vi "Export Test Suite.vi"(8 "error in (no error)":errorcluster, 10 "Test Suite":T1, 11 "Node in":refnum<k20>) -> (0 "error out":errorcluster, 3 "Node out":refnum<k20>)   [LabVIEW 2013, in "JUnit for Azure Pipelines.lvclass"]
uses:
  JUnit for Azure Pipelines.lvclass
  Test Suite.ctl
  Test Case.ctl
  Test Result.ctl
  Test Case Property.ctl
  <vilib>/xml/Close Reference(Node).vi
  <vilib>/xml/NI_XML.lvlib
  XML/XML.lvlib
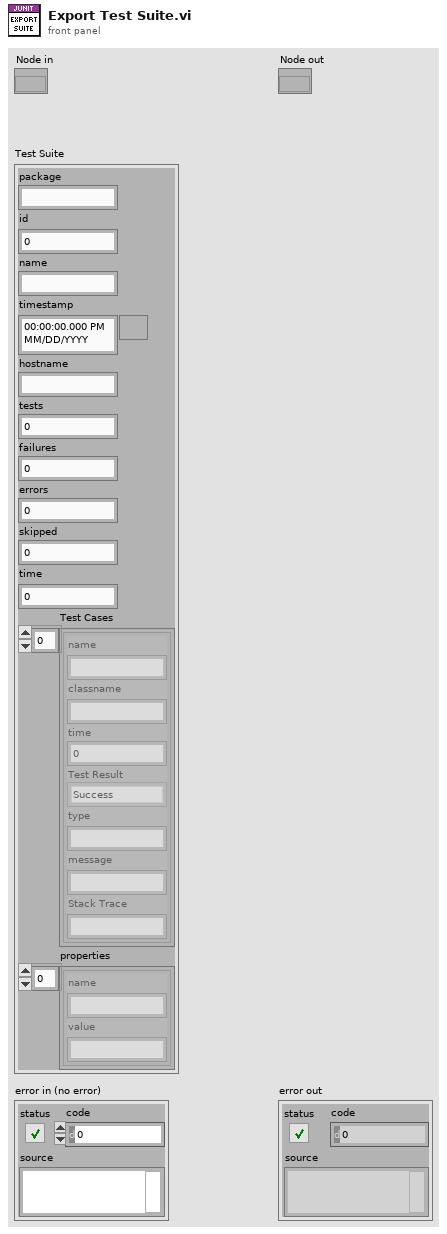
[diagram p1: front panel]
types:
  T1 = typedef "JUnit for Azure Pipelines.lvclass/Test Suite.ctl" = cluster{"package":string, "id":i32, "name":string, "timestamp":timestamp, "hostname":string, "tests":i32, "failures":i32, "errors":i32, "skipped":i32, "time":dbl, "Test Cases":T2[], "properties":T4[]}
  T2 = typedef "JUnit for Azure Pipelines.lvclass/Test Case.ctl" = cluster{"name":string, "classname":string, "time":dbl, "Test Result":T3, "type":string, "message":string, "Stack Trace":string}
  T3 = typedef "JUnit for Azure Pipelines.lvclass/Test Result.ctl" = enum16{"Success", "Failure", "Error", "Skipped"}
  T4 = typedef "JUnit for Azure Pipelines.lvclass/Test Case Property.ctl" = cluster{"name":string, "value":string}
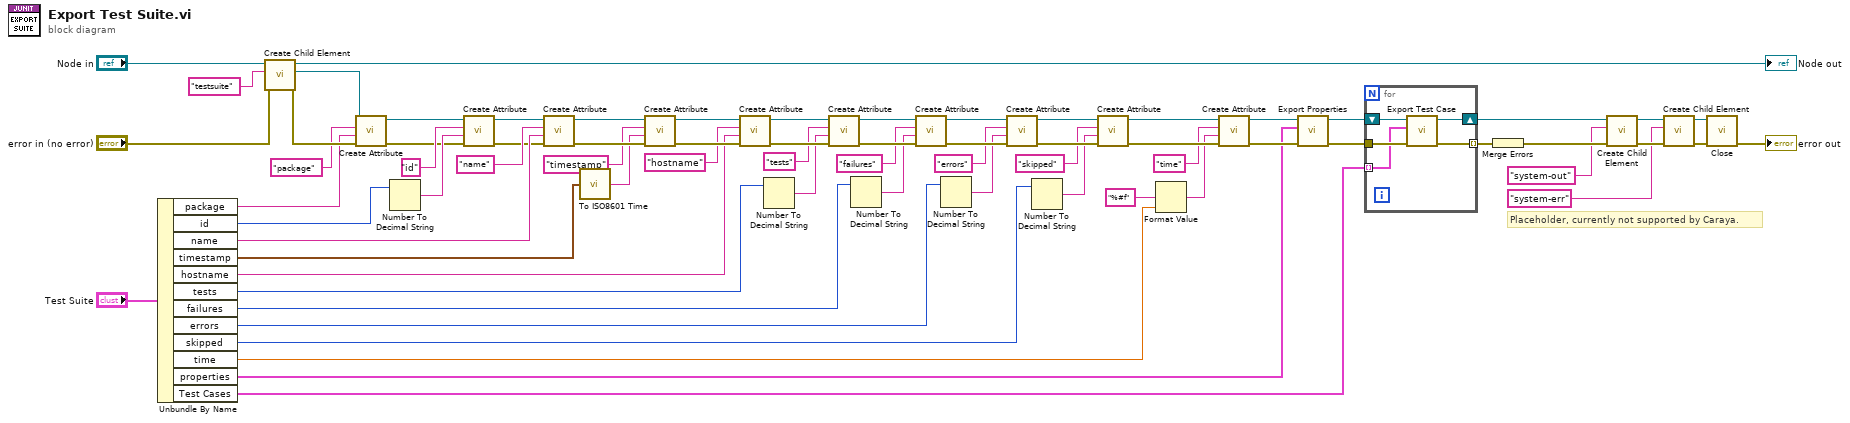
[diagram p0: block diagram]
diagram:
  # "Placeholder, currently not supported by Caraya."
  n1 = Unbundle By Name("Test Suite") -> ("package"=w14:string, "id"=w27:i32, "name"=w62:string, "timestamp"=w58:timestamp, "hostname"=w26:string, "tests"=w25:i32, "failures"=w24:i32, "errors"=w23:i32, "skipped"=w22:i32, "time"=w28:dbl, "properties"=w9:T4[], "Test Cases"=w20:T2[])
  n2 = call "Create Child Element.vi"("error in (no error)"="error in (no error)", "Name"="testsuite" ("Tag Name"), "Element in"="Node in") -> ("error out"=w18:errorcluster, "Child Element"=w17:refnum<k20>, "Element out"=→"Node out":refnum<k20>)  [unwired: 6 in]
  n3 = call "Create Attribute.vi"("error in (no error)"=w18, "Value"=w14, "Name"="package" ("Attribute Name"), "Element in"=w17) -> ("error out"=w19:errorcluster, "Element out"=w16:refnum<k20>)  [unwired: 6 in]
  n4 = Number To Decimal String(number=w27) -> (decimal integer string=w29:string)  [unwired: 1 in]
  n5 = call "Create Attribute.vi"("error in (no error)"=w19, "Value"=w29, "Name"="id" ("Attribute Name"), "Element in"=w16) -> ("error out"=w32:errorcluster, "Element out"=w31:refnum<k20>)  [unwired: 6 in]
  n6 = call "Create Attribute.vi"("error in (no error)"=w32, "Value"=w62, "Name"="name" ("Attribute Name"), "Element in"=w31) -> ("error out"=w60:errorcluster, "Element out"=w61:refnum<k20>)  [unwired: 6 in]
  n7 = call "To ISO8601 Time.vi"("Time Stamp"=w58) -> ("String"=w57:string)  [unwired: 1 in]
  n8 = call "Create Attribute.vi"("error in (no error)"=w60, "Value"=w57, "Name"="timestamp" ("Attribute Name"), "Element in"=w61) -> ("error out"=w55:errorcluster, "Element out"=w56:refnum<k20>)  [unwired: 6 in]
  n9 = call "Create Attribute.vi"("error in (no error)"=w55, "Value"=w26, "Name"="hostname" ("Attribute Name"), "Element in"=w56) -> ("error out"=w52:errorcluster, "Element out"=w53:refnum<k20>)  [unwired: 6 in]
  n10 = Number To Decimal String(number=w25) -> (decimal integer string=w50:string)  [unwired: 1 in]
  n11 = call "Create Attribute.vi"("error in (no error)"=w52, "Value"=w50, "Name"="tests" ("Attribute Name"), "Element in"=w53) -> ("error out"=w49:errorcluster, "Element out"=w48:refnum<k20>)  [unwired: 6 in]
  n12 = Number To Decimal String(number=w24) -> (decimal integer string=w46:string)  [unwired: 1 in]
  n13 = call "Create Attribute.vi"("error in (no error)"=w49, "Value"=w46, "Name"="failures" ("Attribute Name"), "Element in"=w48) -> ("error out"=w44:errorcluster, "Element out"=w45:refnum<k20>)  [unwired: 6 in]
  n14 = Number To Decimal String(number=w23) -> (decimal integer string=w42:string)  [unwired: 1 in]
  n15 = call "Create Attribute.vi"("error in (no error)"=w44, "Value"=w42, "Name"="errors" ("Attribute Name"), "Element in"=w45) -> ("error out"=w40:errorcluster, "Element out"=w41:refnum<k20>)  [unwired: 6 in]
  n16 = Number To Decimal String(number=w22) -> (decimal integer string=w38:string)  [unwired: 1 in]
  n17 = call "Create Attribute.vi"("error in (no error)"=w40, "Value"=w38, "Name"="skipped" ("Attribute Name"), "Element in"=w41) -> ("error out"=w36:errorcluster, "Element out"=w37:refnum<k20>)  [unwired: 6 in]
  n18 = Format Value(format string="%#f", value (0)=w28) -> (output string=w33:string)  [unwired: 1 in]
  n19 = call "Create Attribute.vi"("error in (no error)"=w36, "Value"=w33, "Name"="time" ("Attribute Name"), "Element in"=w37) -> ("error out"=w11:errorcluster, "Element out"=w13:refnum<k20>)  [unwired: 6 in]
  n20 = call "Export Properties.vi"("error in (no error)"=w11, "Properties"=w9, "Node in"=w13) -> ("error out"=w10:errorcluster, "Node out"=w12:refnum<k20>)  [unwired: 7 in]
  n21 = for {
    tunnel: [w72] -> w21 mode=indexing
    tunnel: w10 -> [w71]
    shift-right: [w73] -> w8
    shift-left: w12 -> [w74]
    tunnel: w20 -> [w70] mode=indexing
    n22 = call "Export Test Case.vi"("error in (no error)"=w71, "Test Case"=w70, "Node in"=w74) -> ("error out"=w72:errorcluster, "Node out"=w73:refnum<k20>)  [unwired: 7 in]
  }
  n23 = Merge Errors(w21) -> (w7:errorcluster)
  n24 = call "Create Child Element.vi"("error in (no error)"=w7, "Name"="system-out" ("Tag Name"), "Element in"=w8) -> ("error out"=w5:errorcluster, "Element out"=w6:refnum<k20>)  [unwired: 6 in, 1 out]
  n25 = call "Create Child Element.vi"("error in (no error)"=w5, "Name"="system-err" ("Tag Name"), "Element in"=w6) -> ("error out"=w4:errorcluster, "Element out"=w3:refnum<k20>)  [unwired: 6 in, 1 out]
  n26 = call-poly <vilib>:"Close.vi"("error in (no error)"=w4, "node"=w3) -> ("error out"=→"error out":errorcluster)  [unwired: 7 in]
